vi "BotSpeak_DIOWrite.vi"(0 "State":enum32{"LO", "HI"}(ring)=enum."HI", 2 "Bot Settings":T1, 3 "DIO Line":u32) -> (1 "response":string, 4 "Bot Settings":T1)   [LabVIEW 2012]
doc: "Writes the specified \"State\" (High or Low enumerated constant) to the specified \"DIO Line\""
uses:
  <userlib>/BotSpeak/VIs/Direct/BotSpeak_Control.ctl
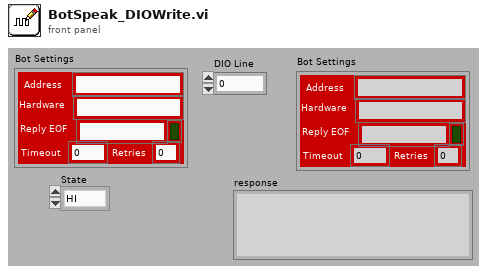
[diagram p1: front panel]
types:
  T1 = typedef "BotSpeak_Control.ctl" = cluster{"Address":string, "Reply EOF":string, "Hardware":string, "Retries":i8, "Timeout":i32, "Open?":bool}
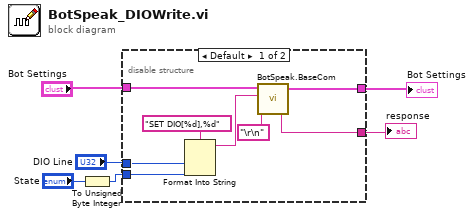
[diagram p0: block diagram]
diagram:
  n1 = To Unsigned Byte Integer(number="State") -> (unsigned 8bit integer=w4:u8)
  n2 = disable-structure shown="Default" {
    disable-tunnel: [w13 _] -> w5
    disable-tunnel: w4 -> [w12 _]
    disable-tunnel: "DIO Line" -> [w11 _]
    disable-tunnel: "Bot Settings" -> [w8 _]
    disable-tunnel: [w7 _] -> w1
    frame condition #0 (active) {
      n3 = Format Into String(format string="SET DIO[%d],%d" ("command"), w11, w12) -> (resulting string=w9:string)  [unwired: 2 in, 1 out]
      n4 = call <userlib>:"BotSpeak.BaseCom.vi"("Termination"="\r\n", "command"=w9, "Bot Settings in"=w8) -> ("response"=w13:string, "Bot Settings out"=w7:T1)  [unwired: 2 in]
    }
    frame condition #1 {
    }
  }
  "response" <- w5
  "Bot Settings" <- w1
